vi "Draw Poly Lines (ARGB).vi"(4 "Draw Mode (Default: Close Points)":T1, 5 "Thickness (Default: 1)":i32=1, 6 "OpenCV Line Type (Default LINE_8)":T5=enum."LINE_8", 7 "ARGB Colour":T4={"Alpha"=255, "RGB"=0}, 8 "error in (no error)":errorcluster, 10 "Points":T2[](array[typedef]), 11 "ARGB Image":T3) -> (0 "error out":errorcluster, 3 "ARGB Image (Duplicate)":T3)   [LabVIEW 2020, in "g_ar_toolkit.image.lvlib"]
uses:
  g_ar_toolkit.image.lvlib
  Line Type.ctl
  ARGB Image.ctl
  ARGB Colour.ctl
  g_ar_toolkit.common/Image Point (Integer).ctl
  Poly Lines Shape Draw Mode.ctl
  f4fe866f-059f-471d-887d-2797bd4b3b13.vi
  g_ar_toolkit.common/Module Path.vi
  <vilib>/Utility/error.llb/Error Cluster From Error Code.vi
  g_ar_toolkit.common/g_ar_toolkit.common.lvlib
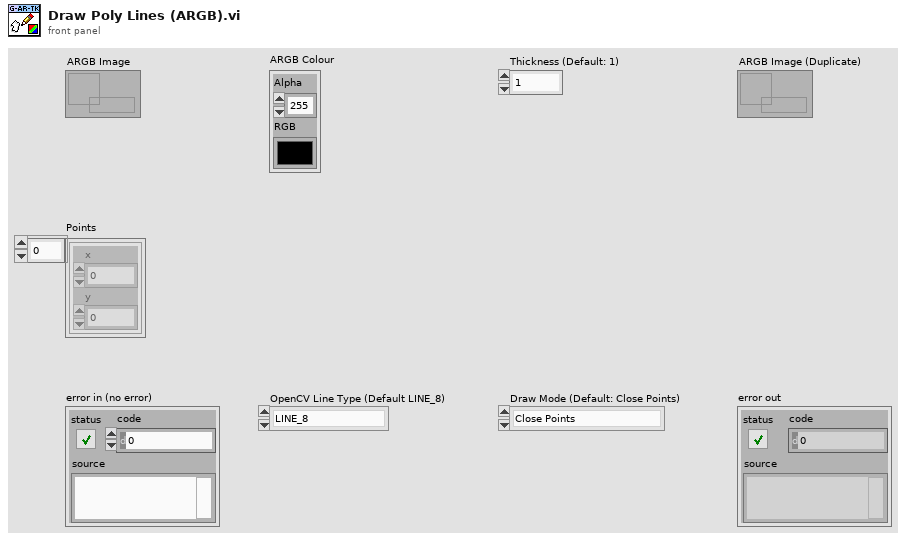
[diagram p1: front panel]
types:
  T1 = typedef "g_ar_toolkit.image.lvlib/Poly Lines Shape Draw Mode.ctl" = enum8{"Close Points", "Leave Points Open"}
  T2 = typedef "g_ar_toolkit.common.lvlib/Image Point (Integer).ctl" = cluster{"x":i32, "y":i32}
  T3 = typedef "g_ar_toolkit.image.lvlib/ARGB Image.ctl" = refnum<data-value>
  T4 = typedef "g_ar_toolkit.image.lvlib/ARGB Colour.ctl" = cluster{"Alpha":u8, "RGB":u32}
  T5 = typedef "g_ar_toolkit.image.lvlib/Line Type.ctl" = enum8{"FILLED", "LINE_4", "LINE_8", "LINE_AA"}
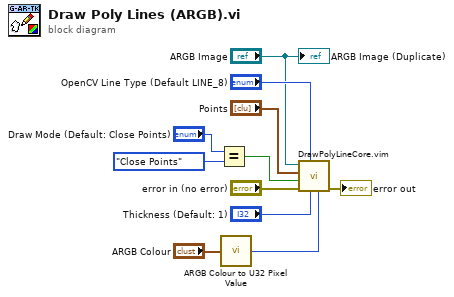
[diagram p0: block diagram]
diagram:
  n1 = Equal?(x="Draw Mode (Default: Close Points)", y=Poly_Lines_Shape_Draw_Mode."Close Points") -> (x = y?=w1:bool)
  n2 = call "ARGB Colour to U32 Pixel Value.vi"("ARGB Colour"="ARGB Colour") -> ("U32 Colour"=w6:u32)
  n3 = call "DrawPolyLineCore.vim"("Colour"=w6, "Thickness"="Thickness (Default: 1)", "OpenCV Line Type"="OpenCV Line Type (Default LINE_8)", "error in (no error)"="error in (no error)", "Is Closed"=w1, "Points"="Points", "Src"="ARGB Image") -> ("error out"=→"error out":errorcluster)  [unwired: 4 in]
  "ARGB Image (Duplicate)" <- "ARGB Image"
